vi "convert rect.vi"(0 "Array Position":cluster{"Row":i32, "Column":i32}) -> (1 "Output Rect":T1, 2 "Output Center":cluster{"Center X":i32, "Center Y":i32})   [LabVIEW 2009]
panel:
  in  "Input Cluster":cluster{"Center X":i32, "Center Y":i32}
  in  "Input Rect Name":T1
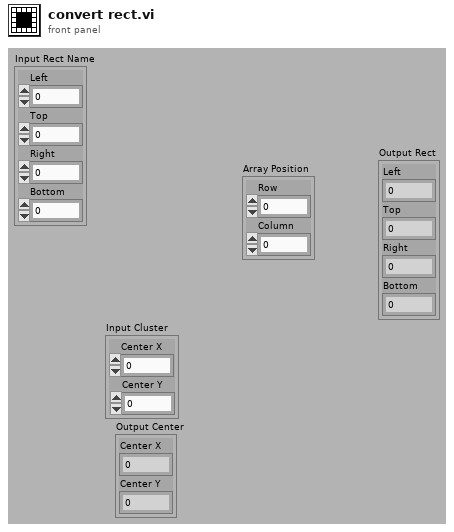
[diagram p1: front panel]
types:
  T1 = cluster{"Left":i32, "Top":i32, "Right":i32, "Bottom":i32}
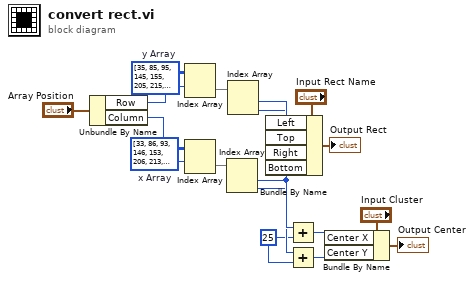
[diagram p0: block diagram]
diagram:
  w5 = 25 ("y")
  w15 = i32[][] [[33, 86], [93, 146], [153, 206], [213, 266], [273, 326], [333, 386], [393, 446], [453, 506], [513, 566], [-1000, 1000]]  # x Array
  w17 = i32[][] [[35, 85], [95, 145], [155, 205], [215, 265], [275, 325], [335, 385], [395, 445], [455, 505], [515, 565], [575, 625], [-1000, 1000]]  # y Array
  n1 = Unbundle By Name("Array Position") -> ("Row"=w16:i32, "Column"=w14:i32)
  n2 = Index Array(array=w17, index (row)=w16) -> (element=w13:i32[])  [unwired: 1 in]
  n3 = Index Array(array=w15, index (row)=w14) -> (element=w12:i32[])  [unwired: 1 in]
  n4 = Index Array(array=w12) -> (element #1=w10:i32, element #2=w9:i32)  [unwired: 2 in]
  n5 = Index Array(array=w13) -> (element #1=w8:i32, element #2=w7:i32)  [unwired: 2 in]
  n6 = Bundle By Name(cluster="Input Rect Name", "Left"=w10, "Top"=w8, "Right"=w9, "Bottom"=w7) -> (→"Output Rect":T1)
  n7 = Add(x=w10, y=w5) -> (x+y=w3:i32)
  n8 = Add(x=w8, y=w5) -> (x+y=w2:i32)
  n9 = Bundle By Name(cluster="Input Cluster", "Center X"=w3, "Center Y"=w2) -> (→"Output Center":cluster{"Center X":i32, "Center Y":i32})
